vi "Time Estimate.vi"(8 "error in (no error)":errorcluster, 9 "expmode":i32, 10 "scantype":T1(ring), 11 "Magnetic Field.lvclass":refnum<class "Magnetic Field.lvclass">) -> (0 "error out":errorcluster, 1 "Time Estimate":string, 2 "time":dbl[unit], 3 "Magnetic Field.lvclass out":refnum<class "Magnetic Field.lvclass">)   [LabVIEW 2009, in "Magnetic Field.lvclass"]
uses:
  Magnetic Field.lvclass
  Global/Set Up.vi
  Magnetic Field.lvclass/Magnetic Field.ctl
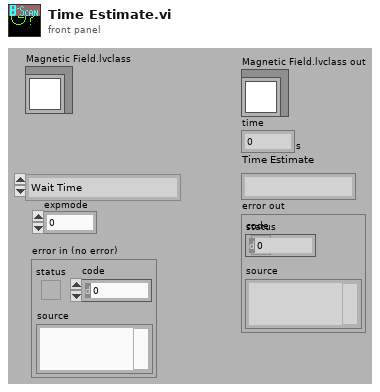
[diagram p1: front panel]
types:
  T1 = enum16{"Wait Time", "Pulse Width", "Wavelength", "Magnetic Field", "rf Scan"}
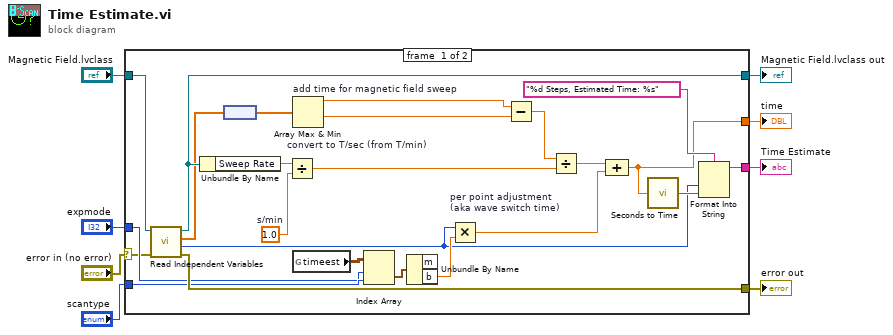
[diagram p0: block diagram]
diagram:
  n1 = case shown="No Error" "error in (no error)" {
    selector: "error in (no error)" -> [w10 w33]
    tunnel: [w12 _] -> w1
    tunnel: "scantype" -> [w27 _]
    tunnel: [w9 _] -> w7
    tunnel: [w28 w34] -> w8
    tunnel: "Magnetic Field.lvclass" -> [w11 w34]
    tunnel: [w29 w33] -> w6
    tunnel: "expmode" -> [w18 _]
    frame #0 {
      w22 = dbl[unit] 1.0  # s/min
      n2 = call-dynamic "Read Independent Variables.vi"("error in (no error)"=w10, "Scanner.lvclass in"=w11) -> ("error out"=w29:errorcluster, "size"=w13:i32, "Independent Variables"=w26:dbl[], "Scanner.lvclass out"=w28:refnum<class "Magnetic Field.lvclass">)  [unwired: 6 out]
      n3 = Unbundle By Name(w28) -> ("Sweep Rate"=w25:dbl[unit])
      n4 = node(w26) -> (w17:dbl[unit][])
      n5 = Divide "convert to T/sec (from T/min)"(x=w25, y=w22) -> (x/y=w23:dbl[unit])
      n6 = Array Max & Min "add time for magnetic field sweep"(array=w17) -> (max value=w20:dbl[unit], min value=w21:dbl[unit])  [unwired: 2 out]
      n7 = global read "Set Up.vi" "timeest"() -> (w32:cluster{"m":dbl, "b":dbl[unit]}[][])
      n8 = Index Array(array=w32, index (row)=w18, index (col)=w27) -> (element=w31:cluster{"m":dbl, "b":dbl[unit]})
      n9 = Unbundle By Name(w31) -> ("b"=w30:dbl[unit])  [unwired: 1 out]
      n10 = Multiply "per point adjustment\n(aka wave switch time)"(x=w13, y=w30) -> (x*y=w16:dbl[unit])
      n11 = Subtract(x=w20, y=w21) -> (x-y=w19:dbl[unit])
      n12 = Divide(x=w19, y=w23) -> (x/y=w24:dbl[unit])
      n13 = Compound Arithmetic op=ADD(w24, w16) -> (w9:dbl[unit])
      n14 = call "Seconds to Time.vi"("Seconds"=w9) -> ("Time"=w14:string)
      n15 = Format Into String(format string="%d Steps, Estimated Time: %s", w13, w14) -> (resulting string=w12:string)  [unwired: 2 in, 1 out]
    }
    frame #1 {
    }
  }
  "time" <- w7
  "Magnetic Field.lvclass out" <- w8
  "error out" <- w6
  "Time Estimate" <- w1
